vi "example-tx-c_api.vi"() -> ()   [LabVIEW 2025]
uses:
  <vilib>/Analysis/1siggen.llb/Ramp Pattern by Samples.vi
  uhd_lv_linux/uhd_imported_fixed/uhd.lvlib
  <vilib>/Analysis/NI_AALBase.lvlib
  <vilib>/measure/NI_MABase.lvlib
panel:
  out "Waveform Graph":waveform(dbl)[](graph)
  in  "waveform size":dbl=10000.0
  in  "amplitude":dbl=0.7 format="%0.2f"
  in  "frequency":dbl=1000.0 format="%0.2p"
  out "ant_out out":string="TX/RX"
  in  "stop":bool
  out "freq_out out":dbl=1000000000.0
  in  "target_freq":dbl=1000000000.0 format="%#_6p"
  in  "ant":string="TX/RX"
  out "gain_out out":dbl
  in  "gain":dbl
  out "rate_out out":dbl=1000000.0
  in  "rate":dbl=1000000.0
  in  "chan":u64
  out "error out":errorcluster
  in  "args":string="addr=10.88.137.205"
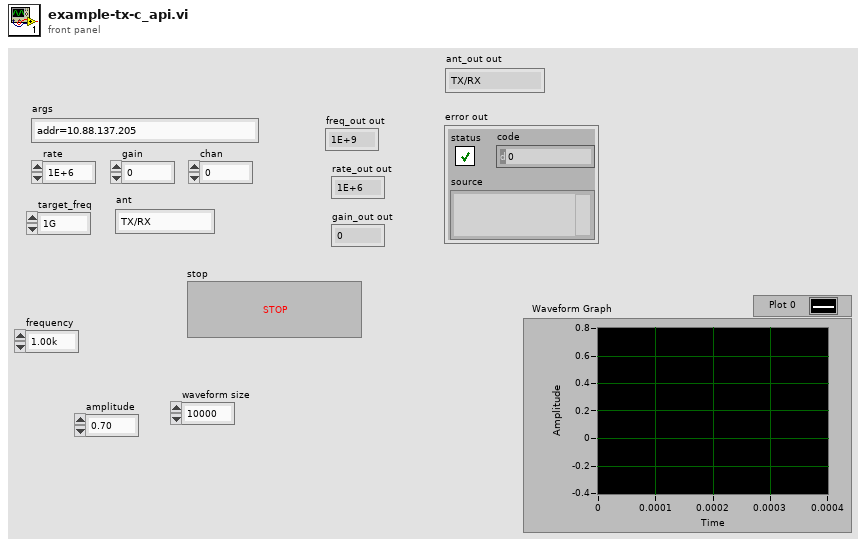
[diagram p1: front panel]
types:
  T1 = cluster{"cpu_format":string, "otw_format":string, "args":string, "channel_list":u64[], "n_channels":u64}
  T2 = cluster{"target_freq":dbl, "rf_freq_policy":u32, "@dummy control@":i8, "@dummy control@":i8, "@dummy control@":i8, "@dummy control@":i8, "rf_freq":dbl, "dsp_freq_policy":u32, "@dummy control@":i8, "@dummy control@":i8, "@dummy control@":i8, "@dummy control@":i8, "dsp_freq":dbl, "args":u64}
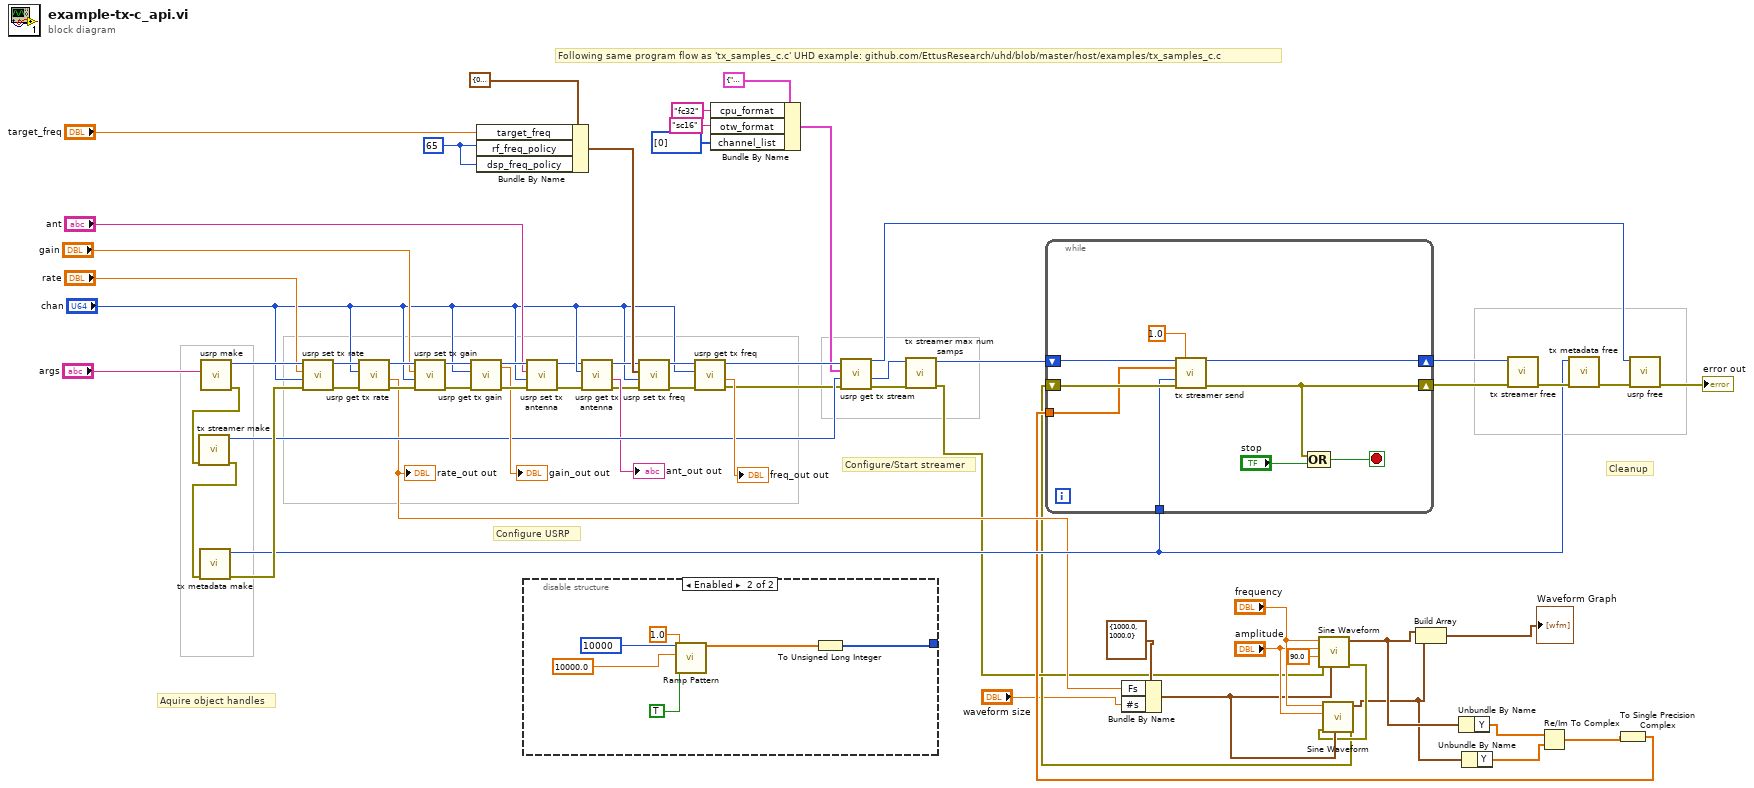
[diagram p0: block diagram]
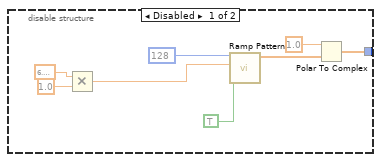
[diagram p2: hidden frame]
diagram:
  w34 = u32 65 ("rf_freq_policy")
  # "Cleanup"
  # "Configure/Start streamer"
  # "Configure USRP"
  # "Aquire object handles"
  # "Following same program flow as 'tx_samples_c.c' UHD example: github.com/EttusResearch/uhd/blob/master/host/examples/tx_samples_c.c"
  n1 = call "usrp make.vi"("args"="args") -> ("error out"=w65:errorcluster, "h"=w63:u64)  [unwired: 8 in, 1 out]
  n2 = call "tx streamer make.vi"("error in (no error)"=w65) -> ("error out"=w51:errorcluster, "h out"=w31:u64)  [unwired: 8 in, 1 out]
  n3 = call "tx metadata make.vi"("error in (no error)"=w51) -> ("error out"=w62:errorcluster, "handle out"=w25:u64)  [unwired: 8 in, 1 out]
  n4 = call "usrp set tx rate.vi"("error in (no error)"=w62, "chan"="chan", "rate"="rate", "h"=w63) -> ("error out"=w61:errorcluster, "h 2"=w50:u64)  [unwired: 5 in, 1 out]
  n5 = call "usrp get tx rate.vi"("error in (no error)"=w61, "chan"="chan", "h"=w50) -> ("error out"=w60:errorcluster, "rate_out out"=w14:dbl, "h 2"=w49:u64)  [unwired: 5 in, 1 out]
  "rate_out out" <- w14
  n6 = call "usrp set tx gain.vi"("error in (no error)"=w60, "chan"="chan", "gain"="gain", "h"=w49) -> ("error out"=w59:errorcluster, "h 2"=w48:u64)  [unwired: 5 in, 1 out]
  n7 = call "usrp get tx gain.vi"("error in (no error)"=w59, "chan"="chan", "h"=w48) -> ("error out"=w58:errorcluster, "h 2"=w47:u64, "gain_out out"=→"gain_out out":dbl)  [unwired: 5 in, 1 out]
  n8 = Bundle By Name(cluster=T2 {"target_freq"=0.0, "rf_freq_policy"=78, "@dummy control@"=0, "@dummy control@"=0, "@dummy control@"=0, "@dummy control@"=0, "rf_freq"=0.0, "dsp_freq_policy"=78, "@dummy control@"=0, "@dummy control@"=0, "@dummy control@"=0, "@dummy control@"=0, "dsp_freq"=0.0, "args"=0} ("tune_request"), "target_freq"="target_freq", "rf_freq_policy"=w34, "dsp_freq_policy"=w34) -> (w33:T2)
  n9 = disable-structure shown="Enabled" {
    disable-tunnel: [w66 w74] -> _
    frame Disabled {
      n10 = Multiply(x=6.283185307179586, y=1.0) -> (x*y=w69:dbl)
      n11 = call-poly <vilib>:"Ramp Pattern.vi"("exclude end?"=TRUE, "end"=w69, "samples"=128) -> ("Ramp Pattern"=w73:dbl[])  [unwired: 7 in, 1 out]
      n12 = Polar To Complex(1:w73, 2:1.0 ("r")) -> (0:w66:cdb[])
    }
    frame Enabled {
      n13 = call-poly <vilib>:"Ramp Pattern.vi"("exclude end?"=TRUE, "start"=1.0, "end"=10000.0, "samples"=10000) -> ("Ramp Pattern"=w75:dbl[])  [unwired: 6 in, 1 out]
      n14 = To Unsigned Long Integer(number=w75) -> (unsigned 32bit integer=w74:u32[])
    }
  }
  n15 = call "usrp set tx antenna.vi"("error in (no error)"=w58, "chan"="chan", "ant"="ant", "h"=w47) -> ("error out"=w21:errorcluster, "h 2"=w22:u64)  [unwired: 5 in, 1 out]
  n16 = call "usrp get tx antenna.vi"("error in (no error)"=w21, "chan"="chan", "h"=w22) -> ("error out"=w19:errorcluster, "ant_out out"=→"ant_out out":string, "h 2"=w24:u64)  [unwired: 5 in, 1 out]
  n17 = call "usrp set tx freq.vi"("error in (no error)"=w19, "chan"="chan", "tune_request"=w33, "h"=w24) -> ("error out"=w57:errorcluster, "h 2"=w46:u64)  [unwired: 2 in, 4 out]
  n18 = call "usrp get tx freq.vi"("error in (no error)"=w57, "chan"="chan", "h"=w46) -> ("error out"=w4:errorcluster, "freq_out out"=→"freq_out out":dbl, "h 2"=w45:u64)  [unwired: 5 in, 1 out]
  n19 = Bundle By Name(cluster=T1 {"cpu_format"="", "otw_format"="", "args"="", "channel_list"=[], "n_channels"=0} ("stream_args 2"), "cpu_format"="fc32", "otw_format"="sc16", "channel_list"=u64[] [0]) -> (w26:T1)
  n20 = call "usrp get tx stream.vi"("error in (no error)"=w4, "tx strm in"=w31, "stream_args"=w26, "h"=w45) -> ("error out"=w56:errorcluster, "tx strm out"=w44:u64, "h 2"=w43:u64)  [unwired: 4 in, 1 out]
  n21 = call "tx streamer max num samps.vi"("error in (no error)"=w56, "h"=w44) -> ("error out"=w3:errorcluster, "h 2"=w42:u64)  [unwired: 6 in, 2 out]
  n22 = Bundle By Name(cluster=cluster{"Fs":dbl, "#s":dbl} {"Fs"=1000.0, "#s"=1000.0} ("sampling info"), "Fs"=w14, "#s"="waveform size") -> (w13:cluster{"Fs":dbl, "#s":dbl})
  n23 = call <vilib>:"Sine Waveform.vi"("sampling info"=w13, "error in (no error)"=w3, "phase"=90.0, "amplitude"="amplitude", "frequency"="frequency") -> ("error out"=w11:errorcluster, "signal out"=w10:waveform(dbl))  [unwired: 5 in]
  n24 = call <vilib>:"Sine Waveform.vi"("sampling info"=w13, "error in (no error)"=w11, "amplitude"="amplitude", "frequency"="frequency") -> ("error out"=w2:errorcluster, "signal out"=w9:waveform(dbl))  [unwired: 6 in]
  n25 = Build Array(w10, w9) -> (→"Waveform Graph":waveform(dbl)[])
  n26 = Unbundle By Name(w10) -> ("Y"=w8:dbl[])
  n27 = Unbundle By Name(w9) -> ("Y"=w7:dbl[])
  n28 = Re/Im To Complex(1:w7, 2:w8) -> (0:w6:cdb[])
  n29 = To Single Precision Complex(1:w6) -> (0:w5:csg[])
  n30 = while {
    shift-right: [w86] -> w41
    shift-left: w42 -> [w87]
    shift-right: [w81] -> w53
    shift-left: w2 -> [w88]
    tunnel: w5 -> [w85]
    tunnel: w25 -> [w83]
    stop <- w80 stop-if-true
    n31 = call "tx streamer send.vi"("h"=w87, "timeout"=1.0, "buffs"=w85, "md"=w83, "error in (no error)"=w88) -> ("h 2"=w86:u64, "error out"=w81:errorcluster)  [unwired: 5 in, 4 out]
    n32 = Compound Arithmetic op=OR(w81, "stop") -> (w80:bool)
  }
  n33 = call "tx streamer free.vi"("error in (no error)"=w53, "h"=w41) -> ("error out"=w54:errorcluster)  [unwired: 7 in, 2 out]
  n34 = call "tx metadata free.vi"("error in (no error)"=w54, "handle"=w25) -> ("error out"=w55:errorcluster)  [unwired: 7 in, 2 out]
  n35 = call "usrp free.vi"("error in (no error)"=w55, "h"=w43) -> ("error out"=→"error out":errorcluster)  [unwired: 7 in, 2 out]
